vi "mod_Trim Burst for Timing.vi"(0 "input complex waveform":T1={"t0"=0.0, "dt"=1.0, "Y"=[]} {"Y" format="%.3f"; "dt" format="%^.2e"; "t0" format="%.4f"}, 5 "upper mask":dbl[](array[numeric]) format="%.2f", 7 "lower mask":dbl[](array[numeric]) format="%.2f", 9 "ideal":dbl[](array[numeric]) format="%.2f", 12 "ideal sync index":i32, 13 "sync found index":dbl format="%.2f") -> (4 "output complex waveform":T1={"t0"=0.0, "dt"=1.0, "Y"=[]} {"Y" format="%.3f"; "dt" format="%^.2e"; "t0" format="%.4f"}, 6 "burst plots":dbl[][](array[numeric]) format="%.2f")   [LabVIEW 2020, in "niDMT.lvlib"]
uses:
  <vilib>/addons/Modulation/niDMT.lvlib
  <vilib>/addons/Modulation/Analog/controls/Complex Data Waveform.ctl
  <vilib>/addons/Modulation/niAMT.lvlib
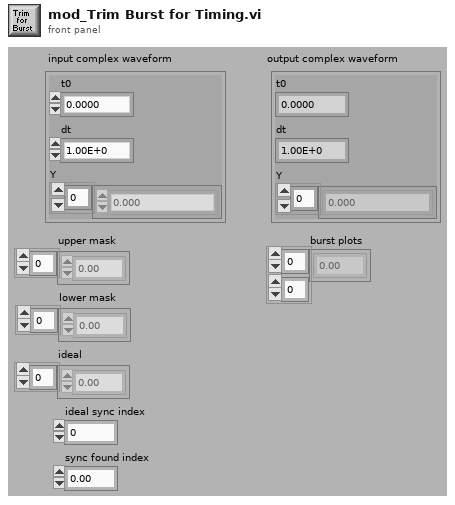
[diagram p1: front panel]
types:
  T1 = typedef "niAMT.lvlib/Complex Data Waveform.ctl" = cluster{"t0":dbl, "dt":dbl, "Y":cdb[]}
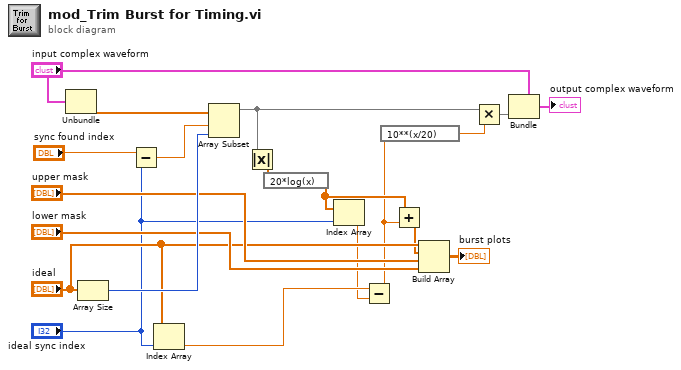
[diagram p0: block diagram]
diagram:
  n1 = Unbundle("input complex waveform") -> ("Y"=w7:cdb[])  [unwired: 2 out]
  n2 = Array Size(array="ideal") -> (size(s)=w20:i32)
  n3 = Subtract(x="sync found index", y="ideal sync index") -> (x-y=w12:dbl)
  n4 = Index Array(array="ideal", index="ideal sync index") -> (element=w9:dbl)
  n5 = Array Subset(array=w7, index=w12, length=w20) -> (w17:cdb[])
  n6 = Absolute Value(x=w17) -> (abs(x)=w14:dbl[])
  n7 = expression code="20*log(x)"(w14) -> (w5:dbl[])
  n8 = Index Array(array=w5, index="ideal sync index") -> (element=w8:dbl)
  n9 = Subtract(x=w9, y=w8) -> (x-y=w3:dbl)
  n10 = expression code="10**(x/20)"(w3) -> (w1:dbl)
  n11 = Add(x=w5, y=w3) -> (x+y=w10:dbl[])
  n12 = Build Array("ideal", w10, "upper mask", "lower mask") -> (→"burst plots":dbl[][])
  n13 = Multiply(x=w17, y=w1) -> (x*y=w2:cdb[])
  n14 = Bundle(cluster="input complex waveform", "Y"=w2) -> (→"output complex waveform":T1)  [unwired: 2 out]
